vi "Update Histogram Data.vi"(10 "Hand String":string, 11 "Histogram In":i32[](array[numeric])) -> (3 "Histogram Out":i32[](array[numeric]))   [LabVIEW 2021]
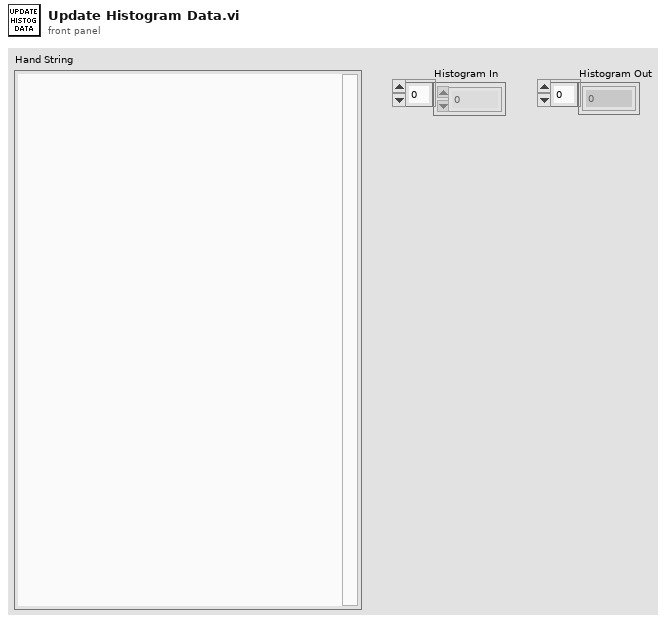
[diagram p1: front panel]
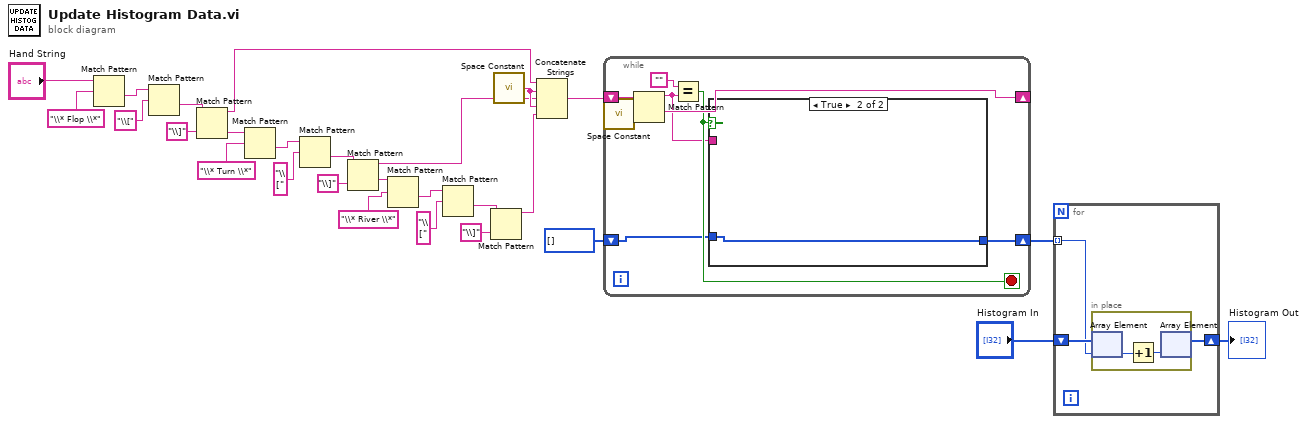
[diagram p0: block diagram]
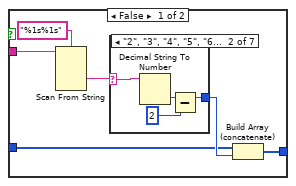
[diagram p2: hidden frame]
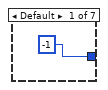
[diagram p3: hidden frame]
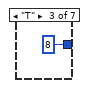
[diagram p4: hidden frame]
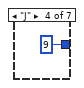
[diagram p5: hidden frame]
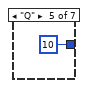
[diagram p6: hidden frame]
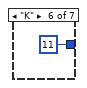
[diagram p7: hidden frame]
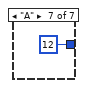
[diagram p8: hidden frame]
diagram:
  n1 = Match Pattern(string="Hand String", regular expression="\\* Flop \\*") -> (after substring=w25:string)  [unwired: 1 in, 3 out]
  n2 = Match Pattern(string=w25, regular expression="\\[") -> (after substring=w23:string)  [unwired: 1 in, 3 out]
  n3 = Match Pattern(string=w23, regular expression="\\]") -> (before substring=w8:string, after substring=w13:string)  [unwired: 1 in, 2 out]
  n4 = Match Pattern(string=w13, regular expression="\\* Turn \\*") -> (after substring=w21:string)  [unwired: 1 in, 3 out]
  n5 = Match Pattern(string=w21, regular expression="\\[") -> (after substring=w19:string)  [unwired: 1 in, 3 out]
  n6 = Match Pattern(string=w19, regular expression="\\]") -> (before substring=w7:string, after substring=w12:string)  [unwired: 1 in, 2 out]
  n7 = Match Pattern(string=w12, regular expression="\\* River \\*") -> (after substring=w17:string)  [unwired: 1 in, 3 out]
  n8 = Match Pattern(string=w17, regular expression="\\[") -> (after substring=w15:string)  [unwired: 1 in, 3 out]
  n9 = Match Pattern(string=w15, regular expression="\\]") -> (before substring=w6:string)  [unwired: 1 in, 3 out]
  n10 = call <vilib>:"Space Constant.vi"() -> ("String"=w9:string)
  n11 = Concatenate Strings(w8, w9, w7, w9, w6) -> (w5:string)
  n12 = while {
    shift-right: [w32] -> _
    shift-left: w5 -> [w35]
    shift-right: [w29] -> w3
    shift-left: i32[] [] -> [w28]
    stop <- w31 stop-if-true
    n13 = call <vilib>:"Space Constant.vi"() -> ("String"=w34:string)
    n14 = Match Pattern(string=w35, regular expression=w34) -> (before substring=w30:string, after substring=w32:string)  [unwired: 1 in, 2 out]
    n15 = Equal?(x="", y=w30) -> (x = y?=w31:bool)
    n16 = case shown="True" w31 {
      tunnel: w30 -> [w41 _]
      tunnel: [w37 w52] -> w29
      tunnel: w28 -> [w36 w52]
      frame False {
        n17 = Scan From String(format string="%1s%1s", input string=w41) -> (output 1=w39:string)  [unwired: 5 in, 3 out]
        n18 = case shown="\"2\", \"3\", \"4\", \"5\", \"6\", \"7\", \"8\", \"9\"" w39 {
          selector: w39 -> [_ w46 _ _ _ _ _]
          tunnel: [-1 w44 8 9 10 11 12] -> w38
          frame Default {
          }
          frame "2", "3", "4", "5", "6", "7", "8", "9" {
            n19 = Decimal String To Number(string=w46) -> (number=w45:i32)  [unwired: 2 in, 1 out]
            n20 = Subtract(x=w45, y=2) -> (x-y=w44:i32)
          }
          frame "T" {
          }
          frame "J" {
          }
          frame "Q" {
          }
          frame "K" {
          }
          frame "A" {
          }
        }
        n21 = Build Array (concatenate)(w36, w38) -> (w37:i32[])
      }
      frame True {
      }
    }
  }
  n22 = for {
    tunnel: w3 -> [w53] mode=indexing
    shift-right: [w54] -> w1
    shift-left: "Histogram In" -> [w55]
    n23 = in-place {
      n24 = in-place-array #1(w55, w53) -> (w57:i32)
      n25 = Increment(x=w57) -> (x+1=w56:i32)
      n26 = in-place-array #1(w56) -> (w54:i32[])  [unwired: 1 out]
    }
  }
  "Histogram Out" <- w1
